vi "MGI Calculate Array Differences (SGL[]).vi"(0 "x(i)":sgl[](array[numeric]) format="%.2f", 1 "x(-1) (default 0)":sgl format="%.2f") -> (2 "y(i)=x(i)-x(i-1)":sgl[](array[numeric]) format="%.2f")   [LabVIEW 2016]
doc: "Calculate differences between consecutive array elements. 0th element of output is equal to x(0)- x(-1), where x(-1) is an optional scalar input that defaults to zero.\n\nAuthored by David A. Moore\nsupport@mooregoodideas.com\nwww.mooregoodideas.com\n\nCopyright (c) 2010, Moore Good Ideas, Inc.\n\nAll rights reserved.\n\nRedistribution and use in source and binary forms, with or without modification, are permitted provided that the following conditions are met:\n\n * Redistributions of source code must retain the above copyright notice, this list of conditions and the following disclaimer.\n * Redistributions in binary form must reproduce the above copyright notice, this list of conditions and the following disclaimer in the documentation and/or other materials provided with the distribution.\n * Neither the name of Moore Good Ideas, Inc. nor the names of its contributors may be used to endorse or promote products derived from this software without specific prior written permission.\n\nTHIS SOFTWARE IS PROVIDED BY THE COPYRIGHT HOLDERS AND CONTRIBUTORS \"AS IS\" AND ANY EXPRESS OR IMPLIED WARRANTIES, INCLUDING, BUT NOT LIMITED TO, THE IMPLIED WARRANTIES OF MERCHANTABILITY AND FITNESS FOR A PARTICULAR PURPOSE ARE DISCLAIMED. IN NO EVENT SHALL THE COPYRIGHT OWNER OR CONTRIBUTORS BE LIABLE FOR ANY DIRECT, INDIRECT, INCIDENTAL, SPECIAL, EXEMPLARY, OR CONSEQUENTIAL DAMAGES (INCLUDING, BUT NOT LIMITED TO, PROCUREMENT OF SUBSTITUTE GOODS OR SERVICES; LOSS OF USE, DATA, OR PROFITS; OR BUSINESS INTERRUPTION) HOWEVER CAUSED AND ON ANY THEORY OF LIABILITY, WHETHER IN CONTRACT, STRICT LIABILITY, OR TORT (INCLUDING NEGLIGENCE OR OTHERWISE) ARISING IN ANY WAY OUT OF THE USE OF THIS SOFTWARE, EVEN IF ADVISED OF THE POSSIBILITY OF SUCH DAMAGE."
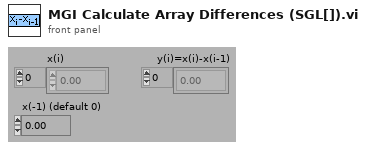
[diagram p1: front panel]
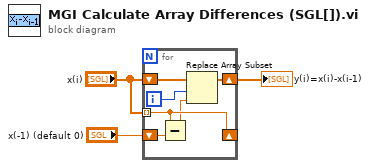
[diagram p0: block diagram]
diagram:
  n1 = for {
    tunnel: "x(i)" -> [w9] mode=indexing
    shift-right: [w9] -> _
    shift-left: "x(-1) (default 0)" -> [w8]
    shift-right: [w6] -> w1
    shift-left: "x(i)" -> [w7]
    i -> [w5]
    n2 = Subtract(x=w9, y=w8) -> (x-y=w4:sgl)
    n3 = Replace Array Subset(array=w7, new element=w4, index=w5) -> (w6:sgl[])
  }
  "y(i)=x(i)-x(i-1)" <- w1
